vi "XML_Get Child Node From Node Name.vi"(8 "error in":errorcluster caption="错误输入（无错误）", 10 "NodeName":string, 11 "ref in":refnum<k20>) -> (0 "错误输出":errorcluster, 1 "find?":bool, 2 "subNode out":refnum<k20>)   [LabVIEW 2016]
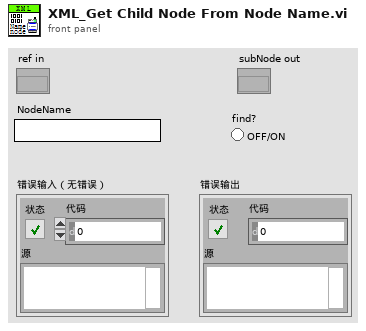
[diagram p1: front panel]
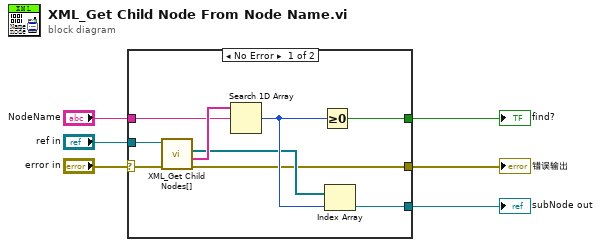
[diagram p0: block diagram]
diagram:
  n1 = case shown="No Error" "error in" {
    selector: "error in" -> [w14 w16]
    tunnel: "ref in" -> [w15 _]
    tunnel: [w8 w16] -> w5
    tunnel: "NodeName" -> [w12 _]
    tunnel: [w11 _] -> w2
    tunnel: [w7 _] -> w1
    frame No Error {
      n2 = call "XML_Get Child Nodes[].vi"("错误输入（无错误）"=w14, "ref in"=w15) -> ("错误输出"=w8:errorcluster, "NodeNames[]"=w13:string[], "ElementChildNod[]"=w9:refnum<k20>[])  [unwired: 6 in, 1 out]
      n3 = Search 1D Array(1D array=w13, element=w12) -> (index of element=w10:i32)  [unwired: 1 in]
      n4 = Greater Or Equal To 0?(x=w10) -> (x >= 0?=w11:bool)
      n5 = Index Array(array=w9, index=w10) -> (element=w7:refnum<k20>)
    }
    frame Error {
    }
  }
  "错误输出" <- w5
  "find?" <- w2
  "subNode out" <- w1
